vi "X_Q_4352.vi"(9 "Type":string) -> (0 "Qn":dbl[](array[numeric]), 2 "L":i32)   [LabVIEW 2015]
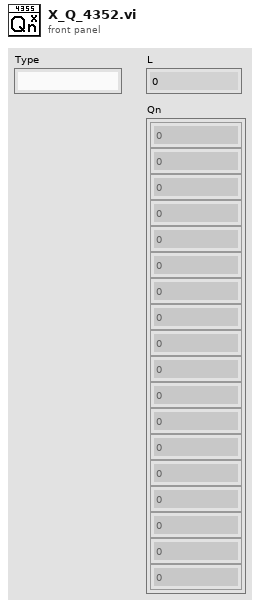
[diagram p1: front panel]
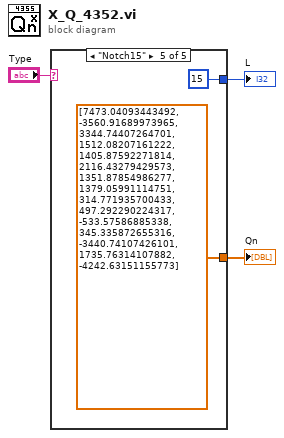
[diagram p0: block diagram]
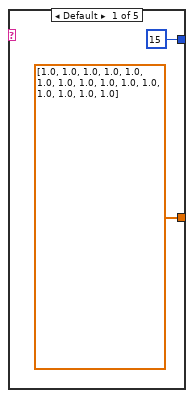
[diagram p2: hidden frame]
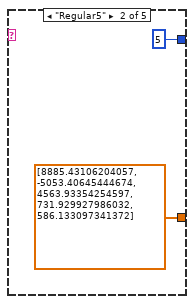
[diagram p3: hidden frame]
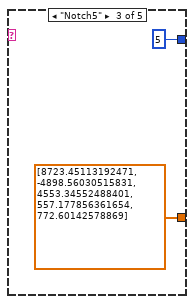
[diagram p4: hidden frame]
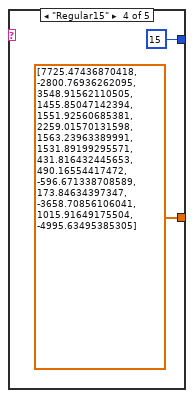
[diagram p5: hidden frame]
diagram:
  n1 = case shown="\"Notch15\"" "Type" {
    tunnel: [15 5 5 15 15] -> w2
    tunnel: [dbl[] [1.0, 1.0, 1.0, 1.0, 1.0, 1.0, 1.0, 1.0, 1.0, 1.0, 1.0, 1.0, 1.0, 1.0, 1.0] ("Qn") dbl[] [8885.43106204057, -5053.40645444674, 4563.93354254597, 731.929927986032, 586.133097341372] ("Qn") dbl[] [8723.45113192471, -4898.56030515831, 4553.34552488401, 557.177856361654, 772.60142578869] ("Qn") dbl[] [7725.47436870418, -2800.76936262095, 3548.91562110505, 1455.85047142394, 1551.92560685381, 2259.01570131598, 1563.23963389991, 1531.89199295571, 431.816432445653, 490.16554417472, -596.671338708589, 173.84634397347, -3658.70856106041, 1015.91649175504, -4995.63495385305] ("Qn") dbl[] [7473.04093443492, -3560.91689973965, 3344.74407264701, 1512.08207161222, 1405.87592271814, 2116.43279429573, 1351.87854986277, 1379.05991114751, 314.771935700433, 497.292290224317, -533.57586885338, 345.335872655316, -3440.74107426101, 1735.76314107882, -4242.63151155773] ("Qn")] -> w1
    frame Default {
    }
    frame "Regular5" {
    }
    frame "Notch5" {
    }
    frame "Regular15" {
    }
    frame "Notch15" {
    }
  }
  "Qn" <- w1
  "L" <- w2
